vi "encodeArrayFloat32.vi"(8 "error in (no error)":errorcluster, 11 "Single Array":sgl[](array[numeric])) -> (0 "error out":errorcluster, 3 "MessagePack":u8[](array[numeric]) format="%.0x")   [LabVIEW 2015, in "MsgPack.lvlib"]
uses:
  MsgPack.lvlib
  encodeFloat32.vi
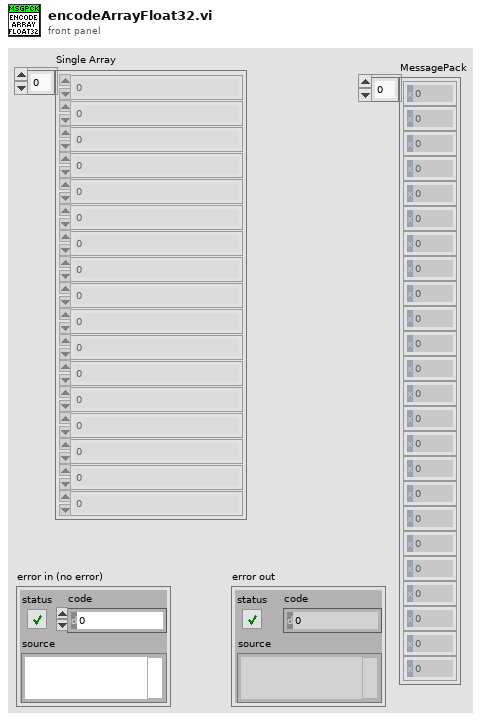
[diagram p1: front panel]
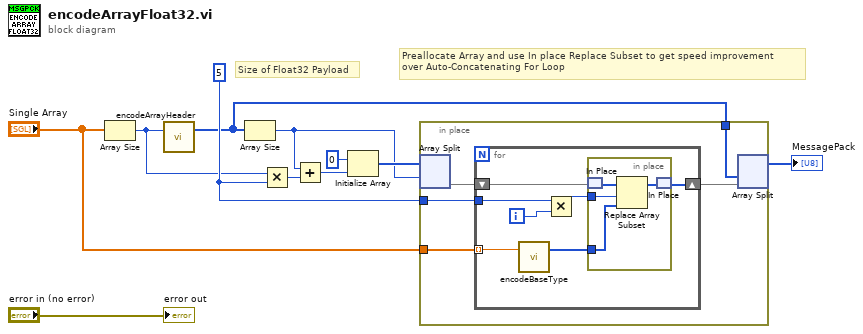
[diagram p0: block diagram]
diagram:
  w6 = 5 ("y")
  # "Preallocate Array and use In place Replace Subset to get speed improvement\nover Auto-Concatenating For Loop"
  # "Size of Float32 Payload"
  n1 = Array Size(array="Single Array") -> (size(s)=w4:i32)
  n2 = call "encodeArrayHeader.vi"("Number of Elements"=w4) -> ("array header"=w2:u8[])  [unwired: 2 in]
  n3 = Array Size(array=w2) -> (size(s)=w7:i32)
  n4 = Multiply(x=w4, y=w6) -> (x*y=w10:i32)
  n5 = Add(x=w7, y=w10) -> (x+y=w9:i32)
  n6 = Initialize Array(u8 0, w9) -> (w8:u8[])
  n7 = in-place {
    in-place-border: w2 -> [w16]
    in-place-border: "Single Array" -> [w15]
    in-place-border: w6 -> [w12]
    n8 = in-place-split #1(w8, w7) -> (w14:u8[])  [unwired: 1 out]
    n9 = for {
      tunnel: w15 -> [w18] mode=indexing
      shift-right: [w22] -> w13
      shift-left: w14 -> [w23]
      tunnel: w12 -> [w20]
      i -> [w21]
      n10 = call-poly "encodeBaseType.vi"("Float32"=w18) -> ("MessagePack"=w17:u8[])  [unwired: 2 in]
      n11 = Multiply(x=w20, y=w21) -> (x*y=w19:i32)
      n12 = in-place {
        in-place-border: w17 -> [w25]
        in-place-border: w19 -> [w24]
        n13 = in-place-match #2(w23) -> (w27:u8[])
        n14 = Replace Array Subset(array=w27, new element=w25, index=w24) -> (w26:u8[])
        n15 = in-place-match #2(w26) -> (w22:u8[])
      }
    }
    n16 = in-place-split #1(w16, w13) -> (→"MessagePack":u8[])  [unwired: 1 out]
  }
  "error out" <- "error in (no error)"
